vi "Aquirer.vi"(8 "Aquirer Index":i32, 9 "Timeout(-1ms)":i32=-1, 10 "Aquirer Queue":refnum<queue>, 11 "Enqueue Lock":T1) -> ()   [LabVIEW 2020, in "Instrument Handler.lvlib" / "Instrument Handler.lvclass"]
doc: "Aquire the Enqueue Lock and send the enqueue the status on the Aquirer Queue."
uses:
  Instrument Handler.lvclass
  Controls/Ctl_AquirerCompletionStatus.ctl
  Instrument Handler.lvlib
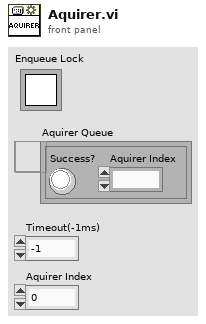
[diagram p1: front panel]
types:
  T1 = typedef "Semaphore RefNum" = refnum<k1>
  T2 = typedef "Instrument Handler.lvlib/Ctl_AquirerCompletionStatus.ctl" = cluster{"Success?":bool, "Aquirer Index":i32}
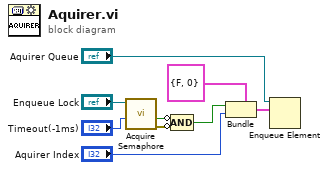
[diagram p0: block diagram]
diagram:
  n1 = call <vilib>:"Acquire Semaphore.vi"("ms timeout (-1)"="Timeout(-1ms)", "semaphore"="Enqueue Lock") -> ("error out"=w5:errorcluster, "timed out"=w6:bool)  [unwired: 3 in, 1 out]
  n2 = Compound Arithmetic op=AND(invert w6, invert w5) -> (w3:bool)
  n3 = Bundle(cluster=T2 {"Success?"=FALSE, "Aquirer Index"=0} ("Instrument cluster"), "Success?"=w3, "Aquirer Index"="Aquirer Index") -> (w1:T2)
  n4 = Enqueue Element(queue="Aquirer Queue", element=w1) -> ()  [unwired: 2 in, 3 out]
